vi "Get Node Info.vi"(8 "error in (no error)":errorcluster, 10 "Active Build Configuration":string, 11 "VIPM Item in":refnum<class "VIPM Item.lvclass">) -> (0 "error out":errorcluster, 1 "Child Nodes":refnum<class "Node.lvclass">[](array[class]), 2 "Label":string)   [LabVIEW 2019, in "VIPM.lvlib" / "VIPM Item.lvclass"]
uses:
  VIPM Item.lvclass
  libs/Solution.lvlibp/Solution/Tree Entry/Node.lvclass
  VIPM Item.lvclass/VIPM Item.ctl
  <vilib>/xml/Close Reference(Node).vi
  <vilib>/xml/Load XML File.vi
  <vilib>/xml/NI_XML.lvlib
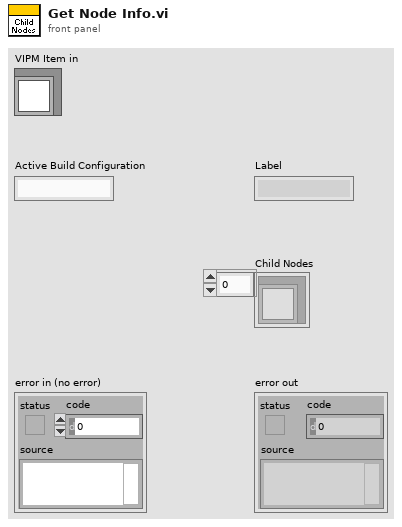
[diagram p1: front panel]
types:
  T1 = typedef "VIPM.lvlib/VIPM Item.lvclass/File Type.ctl" = enum16{"Unsupported", "VIPB", "VIPC"}
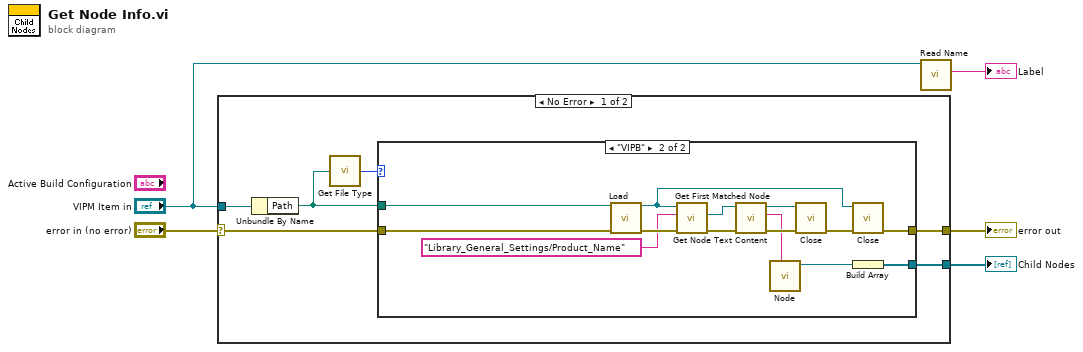
[diagram p0: block diagram]
diagram:
  n1 = case shown="No Error" "error in (no error)" {
    selector: "error in (no error)" -> [w10 w27]
    tunnel: "VIPM Item in" -> [w11 _]
    tunnel: [w9 w27] -> w4
    tunnel: [w6 _] -> w1
    frame No Error {
      n2 = Unbundle By Name(w11) -> ("Path"=w8:path)
      n3 = call "Get File Type.vi"("Path"=w8) -> ("File Type"=w7:T1)  [unwired: 1 in]
      n4 = case shown="\"VIPB\"" w7 {
        tunnel: w10 -> [w12 w19]
        tunnel: [w12 w18] -> w9
        tunnel: w8 -> [_ w17]
        tunnel: [_ w25] -> w6
        frame Default {
        }
        frame "VIPB" {
          n5 = call-poly <vilib>:"Load.vi"("path to XML document"=w17, "error in (no error)"=w19) -> ("DOM document out"=w15:refnum<k20>, "error out"=w24:errorcluster)  [unwired: 11 in, 1 out]
          n6 = call <vilib>:"Get First Matched Node.vi"("error in (no error)"=w24, "XPath expression"="Library_General_Settings/Product_Name", "node in"=w15) -> ("error out"=w22:errorcluster, "node result"=w23:refnum<k20>)  [unwired: 6 in, 1 out]
          n7 = call <vilib>:"Get Node Text Content.vi"("error in (no error)"=w22, "node in"=w23) -> ("error out"=w21:errorcluster, "node text"=w13:string, "node out"=w20:refnum<k20>)  [unwired: 7 in]
          n8 = call "Node.vi"("Name"=w13) -> ("Tree Entry out"=w26:refnum<class "Node.lvclass">)  [unwired: 10 in]
          n9 = call-poly <vilib>:"Close.vi"("error in (no error)"=w21, "node"=w20) -> ("error out"=w14:errorcluster)  [unwired: 7 in]
          n10 = call-poly <vilib>:"Close.vi"("error in (no error)"=w14, "node"=w15) -> ("error out"=w18:errorcluster)  [unwired: 7 in]
          n11 = Build Array(w26) -> (w25:refnum<class "Node.lvclass">[])
        }
      }
    }
    frame Error {
    }
  }
  "error out" <- w4
  "Child Nodes" <- w1
  n12 = call-dynamic "Read Name.vi"("Build Package Item in"="VIPM Item in") -> ("Name"=→"Label":string)  [unwired: 10 in]
